vi "Exit.vi"(8 "error in (no error)":errorcluster, 11 "Image Acquisition in":refnum<class "HAMAMATSU_DCAMAPI.lvclass">) -> (0 "error out":errorcluster, 3 "Image Acquisition out":refnum<class "HAMAMATSU_DCAMAPI.lvclass">)   [LabVIEW 2020, in "HAMAMATSU_DCAMAPI.lvclass"]
uses:
  HAMAMATSU_DCAMAPI.lvclass
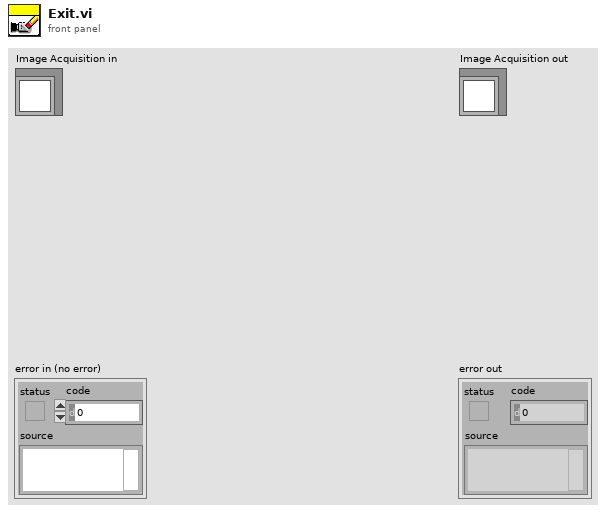
[diagram p1: front panel]
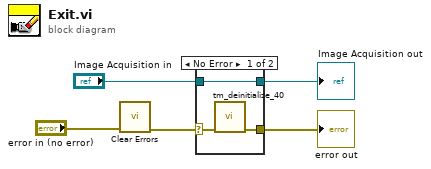
[diagram p0: block diagram]
diagram:
  n1 = call <vilib>:"Clear Errors.vi"("error in (no error)"="error in (no error)") -> ("error out"=w1:errorcluster)  [unwired: 5 in, 1 out]
  n2 = case shown="No Error" w1 {
    selector: w1 -> [w8 w9]
    tunnel: [w7 w9] -> w4
    tunnel: "Image Acquisition in" -> [w6 w10]
    tunnel: [w6 w10] -> w2
    frame No Error {
      n3 = call <userlib>:"tm_deinitialize_40.vi"("error in (no error)"=w8) -> ("error out"=w7:errorcluster)  [unwired: 10 in]
    }
    frame Error {
    }
  }
  "error out" <- w4
  "Image Acquisition out" <- w2
